vi "Cycle_Name.vi"(0 "GEA2 Reference In":refnum<k24>, 11 "error in":errorcluster) -> (4 "GEA2 Reference Out":refnum<k24>, 6 "Cycle Name":string, 15 "error out":errorcluster)   [LabVIEW 2016]
uses:
  Q:/Common/DLLs/GEA3/GeaCommunication.dll
  Common/DLLs/GEA3/GeaCommunication.dll
  Common/LabVIEW GEA2 Toolkit/LabVIEW_GEA2_Toolkit.lvlibp/type defs/Source_Destination.ctl
  Common/LabVIEW GEA2 Toolkit/LabVIEW_GEA2_Toolkit.lvlibp/type defs/ERD Read Data In.ctl
  Common/LabVIEW GEA2 Toolkit/LabVIEW_GEA2_Toolkit.lvlibp/type defs/Data Type.ctl
  Common/LabVIEW GEA2 Toolkit/LabVIEW_GEA2_Toolkit.lvlibp
panel:
  in  "Stand Alone?":bool
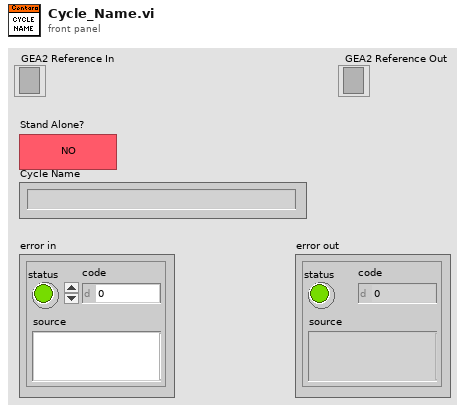
[diagram p1: front panel]
types:
  T1 = typedef "LabVIEW_GEA2_Toolkit.lvlibp/ERD Read Data In.ctl" = cluster{"ERD Number":u16, "Data Type":T2}
  T2 = typedef "LabVIEW_GEA2_Toolkit.lvlibp/Data Type.ctl" = enum16{"string", "boolean", "uint8_t", "uint16_t", "uint32_t", "uint64_t", "int8_t", "int16_t", "int32_t", "int64_t"}
  T3 = typedef "LabVIEW_GEA2_Toolkit.lvlibp/Source_Destination.ctl" = cluster{"Source":u8, "Destination":u8}
  T4 = typedef "LabVIEW_GEA2_Toolkit.lvlibp/ERD Read Data Out.ctl" = cluster{"ERD Number":u16, "Data":string}
  T5 = cluster{"ERD Data Out[0]":T4, "ERD Data Out[1]":T4, "ERD Data Out[2]":T4, "ERD Data Out[3]":T4, "ERD Data Out[4]":T4, "ERD Data Out[5]":T4, "ERD Data Out[6]":T4, "ERD Data Out[7]":T4, "ERD Data Out[8]":T4}
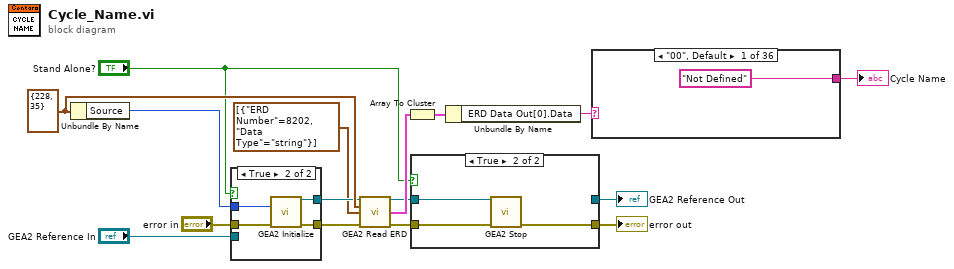
[diagram p0: block diagram]
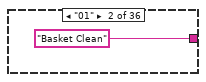
[diagram p4: hidden frame]
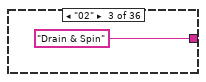
[diagram p5: hidden frame]
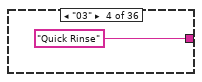
[diagram p6: hidden frame]
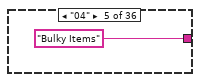
[diagram p7: hidden frame]
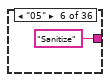
[diagram p8: hidden frame]
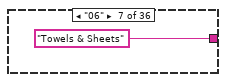
[diagram p9: hidden frame]
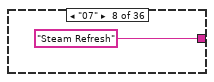
[diagram p10: hidden frame]
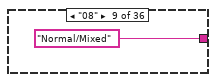
[diagram p11: hidden frame]
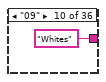
[diagram p12: hidden frame]
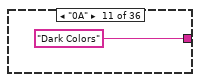
[diagram p13: hidden frame]
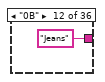
[diagram p14: hidden frame]
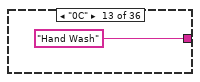
[diagram p15: hidden frame]
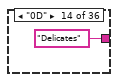
[diagram p16: hidden frame]
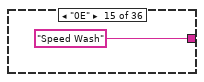
[diagram p17: hidden frame]
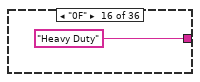
[diagram p18: hidden frame]
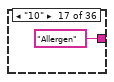
[diagram p19: hidden frame]
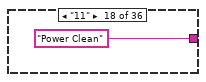
[diagram p20: hidden frame]
diagram:
  w15 = T3 {"Source"=228, "Destination"=35} ("GEA Inputs")
  n1 = Unbundle By Name(w15) -> ("Source"=w14:u8)
  n2 = case shown="True" "Stand Alone?" {
    tunnel: w14 -> [_ w19]
    tunnel: "error in" -> [w17 w22]
    tunnel: "GEA2 Reference In" -> [w18 _]
    tunnel: [w18 w21] -> w11
    tunnel: [w17 w20] -> w10
    frame False {
    }
    frame True {
      n3 = call "GEA2 Initialize.vi"("Source Address"=w19, "error in"=w22) -> ("GEA2 Reference Out"=w21:refnum<k24>, "error out"=w20:errorcluster)  [unwired: 11 in, 1 out]
    }
  }
  n4 = call "GEA2 Read ERD.vi"("GEA2 Reference In"=w11, "GEA Inputs"=w15, "Read ERD List"=T1[] [{"ERD Number"=8202, "Data Type"=enum."string"}], "Error In"=w10) -> ("GEA2 Reference Out"=w5:refnum<k24>, "ERD Data Out"=w8:T4[], "Error Out"=w4:errorcluster)  [unwired: 8 in, 1 out]
  n5 = Array To Cluster(array=w8) -> (cluster=w7:T5)
  n6 = case shown="True" "Stand Alone?" {
    tunnel: w5 -> [w24 w27]
    tunnel: w4 -> [w23 w26]
    tunnel: [w23 w25] -> w3
    tunnel: [w24 _] -> w2
    frame False {
    }
    frame True {
      n7 = call "GEA2 Stop.vi"("GEA2 Reference In"=w27, "Error In"=w26) -> ("Error Out"=w25:errorcluster)  [unwired: 13 in]
    }
  }
  "GEA2 Reference Out" <- w2
  "error out" <- w3
  n8 = Unbundle By Name(w7) -> ("ERD Data Out[0].Data"=w6:string)
  n9 = case shown="\"00\", Default" w6 {
    tunnel: ["Not Defined" "Basket Clean" "Drain & Spin" "Quick Rinse" "Bulky Items" "Sanitize" "Towels & Sheets" "Steam Refresh" "Normal/Mixed" "Whites" "Dark Colors" "Jeans" "Hand Wash" "Delicates" "Speed Wash" "Heavy Duty" "Allergen" "Power Clean" "Rinse & Spin" "Single Item" "Colors" "Cold Wash" "Cottons" "Easy Care" "Active Wear" "Timed Dry" "Dewrinkle" "Air Fluff" "Steam Refresh" "Steam Dewrinkle" "Speed Dry" "Mixed" "Quick Dry" "Casuals" "Warm Up" "Energy Saver"] -> w16
    frame "00", Default {
    }
    frame "01" {
    }
    frame "02" {
    }
    frame "03" {
    }
    frame "04" {
    }
    frame "05" {
    }
    frame "06" {
    }
    frame "07" {
    }
    frame "08" {
    }
    frame "09" {
    }
    frame "0A" {
    }
    frame "0B" {
    }
    frame "0C" {
    }
    frame "0D" {
    }
    frame "0E" {
    }
    frame "0F" {
    }
    frame "10" {
    }
    frame "11" {
    }
    frame "12" {
    }
    frame "13" {
    }
    frame "14" {
    }
    frame "15" {
    }
    frame "80" {
    }
    frame "81" {
    }
    frame "82" {
    }
    frame "83" {
    }
    frame "84" {
    }
    frame "85" {
    }
    frame "86" {
    }
    frame "87" {
    }
    frame "88" {
    }
    frame "89" {
    }
    frame "8A" {
    }
    frame "8B" {
    }
    frame "8C" {
    }
    frame "8D" {
    }
  }
  "Cycle Name" <- w16
